vi "数据状态.vi"(11 "数组":u16[](array[numeric]) format="%04xH") -> (3 "簇":T1)   [LabVIEW 2016, in "一代CodMn.lvlib"]
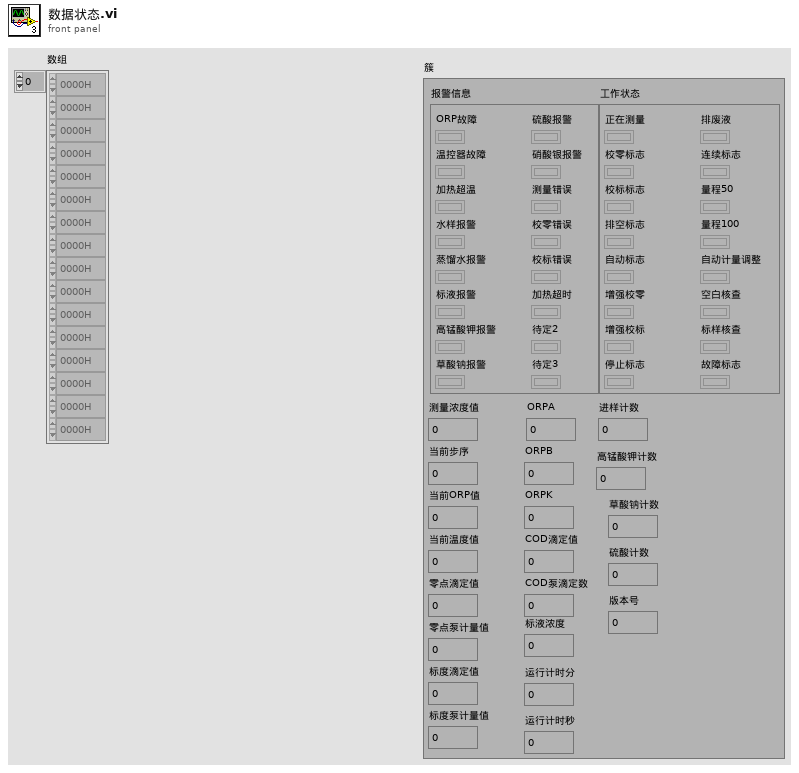
[diagram p1: front panel]
types:
  T1 = cluster{"报警信息":cluster{"ORP故障":bool, "温控器故障":bool, "加热超温":bool, "水样报警":bool, "蒸馏水报警":bool, "标液报警":bool, "高锰酸钾报警":bool, "草酸钠报警":bool, "硫酸报警":bool, "硝酸银报警":bool, "测量错误":bool, "校零错误":bool, "校标错误":bool, "加热超时":bool, "待定2":bool, "待定3":bool}, "工作状态":cluster{"正在测量":bool, "校零标志":bool, "校标标志":bool, "排空标志":bool, "自动标志":bool, "增强校零":bool, "增强校标":bool, "停止标志":bool, "排废液":bool, "连续标志":bool, "量程50":bool, "量程100":bool, "自动计量调整":bool, "空白核查":bool, "标样核查":bool, "故障标志":bool}, "测量浓度值":sgl, "当前步序":u16, "当前ORP值":i16, "当前温度值":sgl, "零点滴定值":sgl, "零点泵计量值":i16, "标度滴定值":sgl, "标度泵计量值":i16, "ORPA":i16, "ORPB":i16, "ORPK":i16, "COD滴定值":sgl, "COD泵滴定数":u16, "标液浓度":sgl, "运行计时分":u16, "运行计时秒":u16, "进样计数":u16, "高锰酸钾计数":u16, "草酸钠计数":u16, "硫酸计数":u16, "版本号":u32}
  T2 = cluster{"报警信息":cluster{"ORP故障":bool, "温控器故障":bool, "加热故障":bool, "水样报警":bool, "蒸馏水报警":bool, "标液报警":bool, "高锰酸钾报警":bool, "草酸钠报警":bool, "硫酸报警":bool, "硝酸银报警":bool, "测量错误":bool, "校零错误":bool, "校标错误":bool, "待定1":bool, "待定2":bool, "待定3":bool}, "工作状态":cluster{"正在测量":bool, "校零标志":bool, "校标标志":bool, "排空标志":bool, "自动标志":bool, "增强校零":bool, "增强校标":bool, "停止标志":bool, "排废液":bool, "连续标志":bool, "量程50":bool, "量程100":bool, "自动计量调整":bool, "空白核查":bool, "标样核查":bool, "故障标志":bool}, "测量浓度值":sgl, "当前步序":u16, "当前ORP值":i16, "当前温度值":sgl, "零点滴定值":sgl, "零点泵计量值":i16, "标度滴定值":sgl, "标度泵计量值":i16, "ORPA":i16, "ORPB":i16, "ORPK":i16, "COD滴定值":sgl, "COD泵滴定数":u16, "标液浓度":sgl, "运行计时分":u16, "运行计时秒":u16, "进样计数":u16, "高锰酸钾计数":u16, "草酸钠计数":u16, "硫酸计数":u16, "版本号":u32}
  T3 = cluster{"Boolean array[0]":bool, "Boolean array[1]":bool, "Boolean array[2]":bool, "Boolean array[3]":bool, "Boolean array[4]":bool, "Boolean array[5]":bool, "Boolean array[6]":bool, "Boolean array[7]":bool, "Boolean array[8]":bool, "Boolean array[9]":bool, "Boolean array[10]":bool, "Boolean array[11]":bool, "Boolean array[12]":bool, "Boolean array[13]":bool, "Boolean array[14]":bool, "Boolean array[15]":bool}
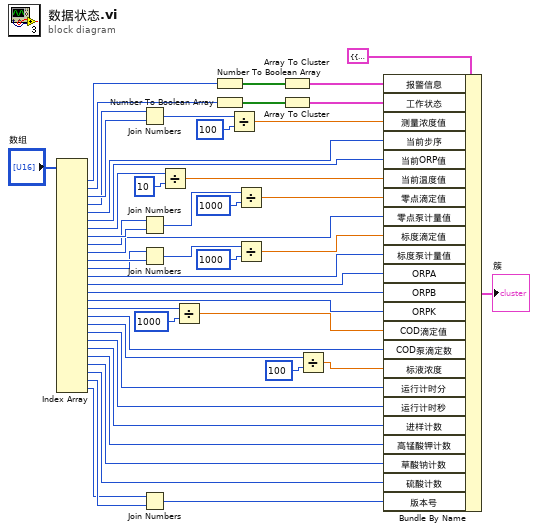
[diagram p0: block diagram]
diagram:
  n1 = Index Array(array="数组") -> (element #1=w49:u16, element #2=w45:u16, element #3=w40:u16, element #4=w39:u16, element #5=w38:u16, element #6=w37:u16, element #7=w35:u16, element #8=w31:u16, element #9=w30:u16, element #10=w28:u16, element #11=w25:u16, element #12=w24:u16, element #13=w22:u16, element #14=w21:u16, element #15=w20:u16, element #16=w19:u16, element #17=w17:u16, element #18=w15:u16, element #19=w13:u16, element #20=w11:u16, element #21=w10:u16, element #22=w9:u16, element #23=w8:u16, element #24=w7:u16, element #25=w6:u16, element #26=w3:u16, element #27=w2:u16)  [unwired: 27 in]
  n2 = Join Numbers(hi=w39, lo=w40) -> ((hi.lo)=w43:u32)
  n3 = Join Numbers(hi=w30, lo=w31) -> ((hi.lo)=w32:u32)
  n4 = Join Numbers(hi=w24, lo=w25) -> ((hi.lo)=w27:u32)
  n5 = Join Numbers(hi=w2, lo=w3) -> ((hi.lo)=w1:u32)
  n6 = Divide(x=w35, y=u32 10) -> (x/y=w34:dbl)
  n7 = Divide(x=w17, y=u32 1000) -> (x/y=w16:dbl)
  n8 = Number To Boolean Array(number=w49) -> (Boolean array=w48:bool[])
  n9 = Number To Boolean Array(number=w45) -> (Boolean array=w46:bool[])
  n10 = Divide(x=w43, y=u32 100) -> (x/y=w41:dbl)
  n11 = Divide(x=w32, y=u32 1000) -> (x/y=w29:dbl)
  n12 = Divide(x=w27, y=u32 1000) -> (x/y=w23:dbl)
  n13 = Array To Cluster(array=w48) -> (cluster=w47:T3)
  n14 = Array To Cluster(array=w46) -> (cluster=w44:T3)
  n15 = Divide(x=w13, y=u32 100) -> (x/y=w12:dbl)
  n16 = Bundle By Name(cluster=T2 {"报警信息"={"ORP故障"=FALSE, "温控器故障"=FALSE, "加热故障"=FALSE, "水样报警"=FALSE, "蒸馏水报警"=FALSE, "标液报警"=FALSE, "高锰酸钾报警"=FALSE, "草酸钠报警"=FALSE, "硫酸报警"=FALSE, "硝酸银报警"=FALSE, "测量错误"=FALSE, "校零错误"=FALSE, "校标错误"=FALSE, "待定1"=FALSE, "待定2"=FALSE, "待定3"=FALSE}, "工作状态"={"正在测量"=FALSE, "校零标志"=FALSE, "校标标志"=FALSE, "排空标志"=FALSE, "自动标志"=FALSE, "增强校零"=FALSE, "增强校标"=FALSE, "停止标志"=FALSE, "排废液"=FALSE, "连续标志"=FALSE, "量程50"=FALSE, "量程100"=FALSE, "自动计量调整"=FALSE, "空白核查"=FALSE, "标样核查"=FALSE, "故障标志"=FALSE}, "测量浓度值"=0.0, "当前步序"=0, "当前ORP值"=0, "当前温度值"=0.0, "零点滴定值"=0.0, "零点泵计量值"=0, "标度滴定值"=0.0, "标度泵计量值"=0, "ORPA"=0, "ORPB"=0, "ORPK"=0, "COD滴定值"=0.0, "COD泵滴定数"=0, "标液浓度"=0.0, "运行计时分"=0, "运行计时秒"=0, "进样计数"=0, "高锰酸钾计数"=0, "草酸钠计数"=0, "硫酸计数"=0, "版本号"=0} ("簇"), "报警信息"=w47, "工作状态"=w44, "测量浓度值"=w41, "当前步序"=w38, "当前ORP值"=w37, "当前温度值"=w34, "零点滴定值"=w29, "零点泵计量值"=w28, "标度滴定值"=w23, "标度泵计量值"=w22, "ORPA"=w21, "ORPB"=w20, "ORPK"=w19, "COD滴定值"=w16, "COD泵滴定数"=w15, "标液浓度"=w12, "运行计时分"=w11, "运行计时秒"=w10, "进样计数"=w9, "高锰酸钾计数"=w8, "草酸钠计数"=w7, "硫酸计数"=w6, "版本号"=w1) -> (→"簇":T2)
